vi "Method.vi"(4 "Value":refnum<class "Abs_Value.lvclass">) -> (1 "Result":refnum<class "ConvertTo_JSON.lvclass">)   [LabVIEW 2021, in "ConvertTo_JSON.lvclass"]
uses:
  ConvertTo_JSON.lvclass
  Abs_Types/Value/Abs_Value.lvclass
  ConvertTo_JSON.lvclass/ConvertTo_JSON.ctl
  Properties/Write Value.vi
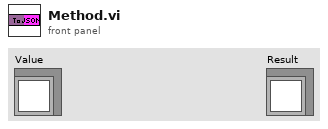
[diagram p1: front panel]
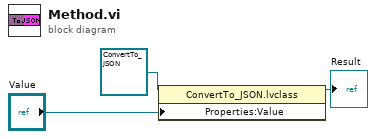
[diagram p0: block diagram]
diagram:
  n1 = property class="ConvertTo_JSON.lvclass"(reference=refnum<class "ConvertTo_JSON.lvclass"> refnum ("ConvertTo_DBL.lvclass"), "Properties:Value"="Value") -> (reference out=→"Result":refnum<class "ConvertTo_JSON.lvclass">)  [unwired: 1 in, 1 out]
